vi "ASI_serialWaitForStatus.vi"(2 "error in":errorcluster, 3 "VISA resource name":refnum<visa-resource-name>="COM1") -> (0 "error out":errorcluster)   [LabVIEW 2015]
doc: "Sends STATUS command every 50 ms up to nStatusTries times.\nIf reply 'N' is received within nStatusTries times, then returns with Success = TRUE,\nelse returns with Success = FALSE."
uses:
  <vilib>/Instr/_visa.llb/VISA Flush IO Buffer Mask.ctl
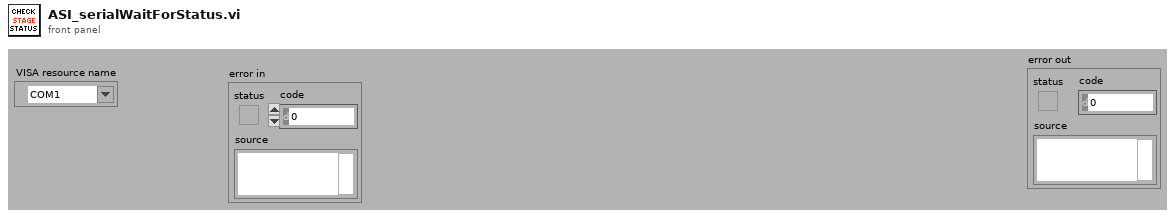
[diagram p1: front panel]
types:
  T1 = typedef "VISA Flush IO Buffer Mask.ctl" = u16
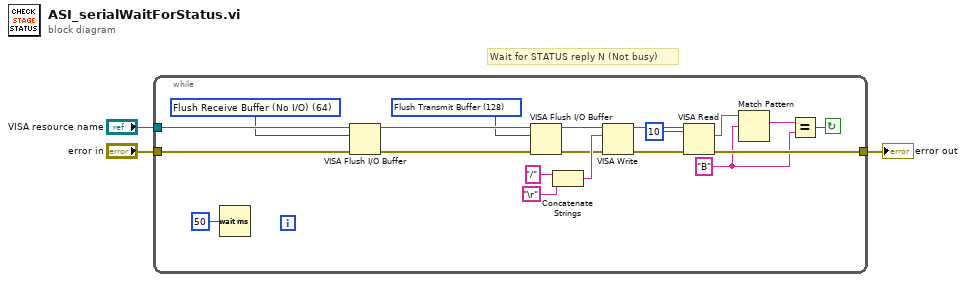
[diagram p0: block diagram]
diagram:
  # "Wait for STATUS reply N (Not busy)"
  n1 = while {
    tunnel: "VISA resource name" -> [w15]
    tunnel: "error in" -> [w14]
    tunnel: [w16] -> w3
    stop <- w4 continue-if-true
    w5 = "B"
    w10 = T1 128 items=["Flush Receive Buffer"=16, "Write Transmit Buffer to Device"=32, "Flush Receive Buffer (No I/O)"=64, "Flush Transmit Buffer"=128] ("Mask")
    w13 = T1 64 items=["Flush Receive Buffer"=16, "Write Transmit Buffer to Device"=32, "Flush Receive Buffer (No I/O)"=64, "Flush Transmit Buffer"=128] ("Mask")
    n2 = Wait (ms)(milliseconds to wait=u32 50) -> ()  [unwired: 1 out]
    n3 = VISA Flush I/O Buffer(VISA resource name=w15, mask (16)=w13, error in (no error)=w14) -> (VISA resource name out=w12:refnum<visa-resource-name>, error out=w11:errorcluster)
    n4 = VISA Flush I/O Buffer(VISA resource name=w12, mask (16)=w10, error in (no error)=w11) -> (VISA resource name out=w8:refnum<visa-resource-name>, error out=w9:errorcluster)
    n5 = Concatenate Strings("/" ("string"), "\r") -> (w21:string)
    n6 = VISA Write(VISA resource name=w8, write buffer=w21, error in (no error)=w9) -> (VISA resource name out=w20:refnum<visa-resource-name>, error out=w18:errorcluster)  [unwired: 1 out]
    n7 = VISA Read(VISA resource name=w20, byte count=u32 10, error in (no error)=w18) -> (read buffer=w7:string, error out=w16:errorcluster)  [unwired: 2 out]
    n8 = Match Pattern(string=w7, regular expression=w5) -> (match substring=w6:string)  [unwired: 1 in, 3 out]
    n9 = Equal?(x=w6, y=w5) -> (x = y?=w4:bool)
  }
  "error out" <- w3
